vi "Toolbar Set Button Image (File).vi"(0 "Display State In":T2={"Buttons Displayed"=0, "Button States"=[], "Button Size"=0, "Button Style"=enum."Classic", "Active Button"=0, "Force Regen?"=FALSE, "Tip String Ref"=refnum}, 1 "Button Index":i32, 5 "State":T1, 7 "Path":path, 9 "Container State":T4, 11 "error in (no error)":errorcluster) -> (4 "Display State Out":T2={"Buttons Displayed"=0, "Button States"=[], "Button Size"=0, "Button Style"=enum."Classic", "Active Button"=0, "Force Regen?"=FALSE, "Tip String Ref"=refnum}, 15 "error out":errorcluster)   [LabVIEW 2012, in "Toolbar.xctl"]
doc: "Set the a specific button's image for a specific state by loading the picture from file. Supports png, bmp and jpeg images."
uses:
  Toolbar.xctl
  <vilib>/_xctls/Container State.ctl
  Toolbar State.ctl
  Button_Class/Button.lvclass
  Button_Class/Type Defs/Button Style.ctl
  Button_Class/Type Defs/Button Status.ctl
  <vilib>/_xctls/XControlSupport.lvlib
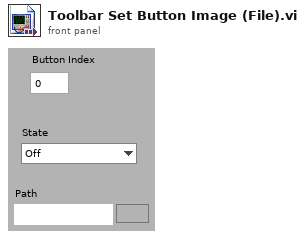
[diagram p1: front panel]
types:
  T1 = typedef "Button.lvclass/Button Status.ctl" = enum16{"Off", "Hover", "On", "Disabled"}
  T2 = typedef "Toolbar.xctl/Toolbar State.ctl" = cluster{"Buttons Displayed":i32, "Button States":refnum<class "Button.lvclass">[], "Button Size":i32, "Button Style":T3, "Active Button":i32, "Force Regen?":bool, "Tip String Ref":refnum<vi>}
  T3 = typedef "Button.lvclass/Button Style.ctl" = enum16{"System", "Modern", "Classic", "Rounded", "Silver", "Ni Theme", "Metallic"}
  T4 = typedef "XControlSupport.lvlib/Container State.ctl" = cluster{"Indicator?":bool, "Run Mode?":bool, " Refnum":refnum<vi>}
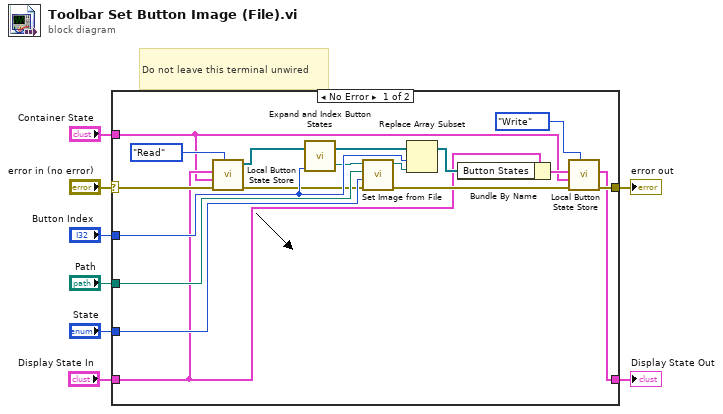
[diagram p0: block diagram]
diagram:
  # "Do not leave this terminal unwired"
  n1 = case shown="No Error" "error in (no error)" {
    selector: "error in (no error)" -> [w19 w27]
    tunnel: "Display State In" -> [w13 w28]
    tunnel: [w11 w28] -> w6
    tunnel: [w14 w27] -> w5
    tunnel: "Button Index" -> [w22 _]
    tunnel: "Path" -> [w26 _]
    tunnel: "State" -> [w25 _]
    tunnel: "Container State" -> [w10 _]
    frame No Error {
      n2 = call "Local Button State Store.vi"("Operation"=enum16{"Read", "Write"}."Read", "error in (no error)"=w19, "Container State"=w10, "Display State In"=w13) -> ("error out"=w18:errorcluster, "Button States"=w9:refnum<class "Button.lvclass">[])  [unwired: 6 out]
      n3 = call "Expand and Index Button States.vi"("Button Index"=w22, "Button States"=w9) -> ("Button.lvclass"=w21:refnum<class "Button.lvclass">, "Button States Out"=w23:refnum<class "Button.lvclass">[])
      n4 = call-dynamic "Set Image from File.vi"("error in (no error)"=w18, "State"=w25, "path"=w26, "Button in"=w21) -> ("error out"=w15:errorcluster, "Button out"=w24:refnum<class "Button.lvclass">)  [unwired: 6 out]
      n5 = Replace Array Subset(array=w23, new element=w24, index=w22) -> (w17:refnum<class "Button.lvclass">[])
      n6 = Bundle By Name(cluster=w13, "Button States"=w17) -> (w12:T2)
      n7 = call "Local Button State Store.vi"("Operation"=enum16{"Read", "Write"}."Write", "error in (no error)"=w15, "Container State"=w10, "Display State In"=w12) -> ("error out"=w14:errorcluster, "Display State Out"=w11:T2)  [unwired: 1 in, 5 out]
    }
    frame Error {
    }
  }
  "Display State Out" <- w6
  "error out" <- w5
